vi "Initialize MeasurementLink Session.vi"(7 "gRPC device options":T1, 8 "error in (no error)":errorcluster, 9 "create session?":bool, 10 "resource name":string, 11 "instrument in":refnum<class "Instrument.lvclass">) -> (0 "error out":errorcluster, 2 "session out":variant, 3 "instrument out":refnum<class "Instrument.lvclass">)   [LabVIEW 2020, in "MeasurementLink Instrument.lvlib" / "Instrument.lvclass"]
doc: "Creates a new session or attaches to an existing session for the provided resource name."
uses:
  Instrument.lvclass
  gRPC Device Options.ctl
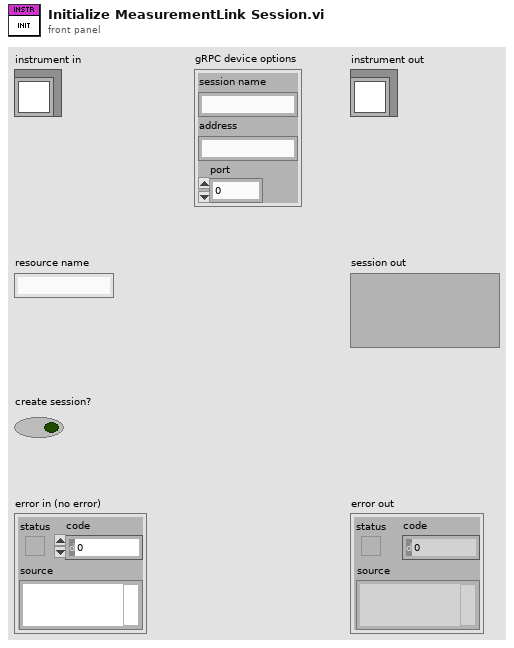
[diagram p1: front panel]
types:
  T1 = typedef "MeasurementLink Instrument.lvlib/Instrument.lvclass/gRPC Device Options.ctl" = cluster{"session name":string, "address":string, "port":i32}
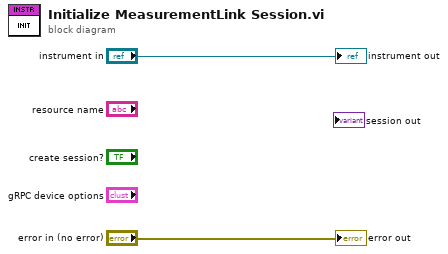
[diagram p0: block diagram]
diagram:
  "error out" <- "error in (no error)"
  "instrument out" <- "instrument in"
